vi "maximize_this.vi"(1 "Phi":dbl, 2 "Goal Angle":dbl, 3 "Theta":dbl) -> (0 "Value":dbl)   [LabVIEW 2011]
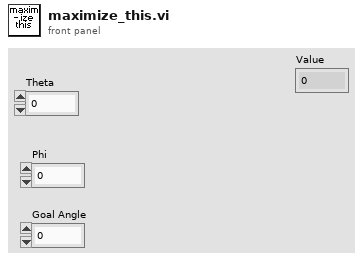
[diagram p1: front panel]
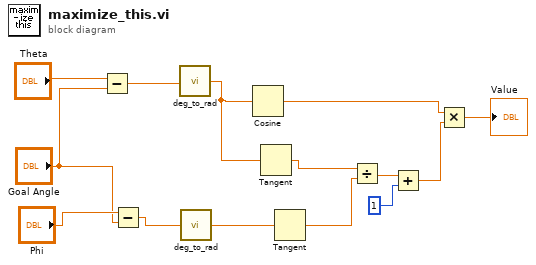
[diagram p0: block diagram]
diagram:
  n1 = Subtract(x="Theta", y="Goal Angle") -> (x-y=w5:dbl)
  n2 = Subtract(x="Phi", y="Goal Angle") -> (x-y=w1:dbl)
  n3 = call "deg_to_rad.vi"("Degrees"=w5) -> ("Radians"=w7:dbl)
  n4 = call "deg_to_rad.vi"("Degrees"=w1) -> ("Radians"=w6:dbl)
  n5 = Cosine(x=w7) -> (cos(x)=w9:dbl)
  n6 = Tangent(1:w7) -> (0:w14:dbl)
  n7 = Tangent(1:w6) -> (0:w13:dbl)
  n8 = Divide(x=w14, y=w13) -> (x/y=w12:dbl)
  n9 = Add(x=w12, y=1) -> (x+y=w10:dbl)
  n10 = Multiply(x=w9, y=w10) -> (x*y=→"Value":dbl)
